vi "hardware_initialize_hardware.vi"(8 "error in (no error)":errorcluster, 11 "tt20 in":refnum<class "tt20.lvclass">) -> (0 "error out":errorcluster, 3 "tt20 out":refnum<class "tt20.lvclass">)   [LabVIEW 2015, in "tt20.lvclass"]
uses:
  tt20.lvclass
  tt20.lvclass/tt20.ctl
  C:/Users/MX-Microscope/Documents/LabVIEW Data/lvoop_campus_2018/Detector_Class/Swabian/time_tagger_vis/TTCSharp32.dll
  time_tagger_vis/TTCSharp32.dll
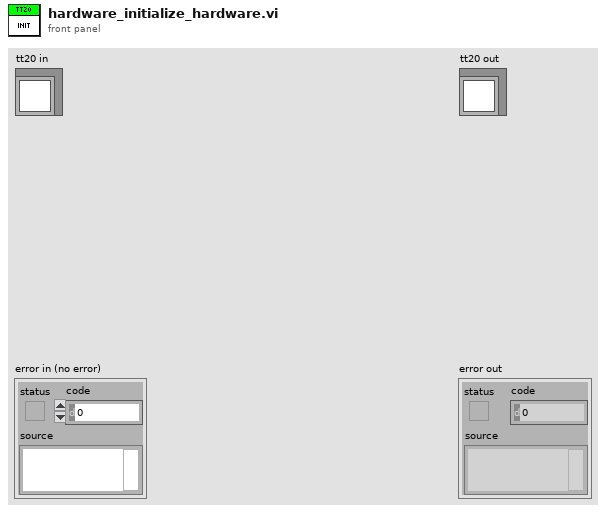
[diagram p1: front panel]
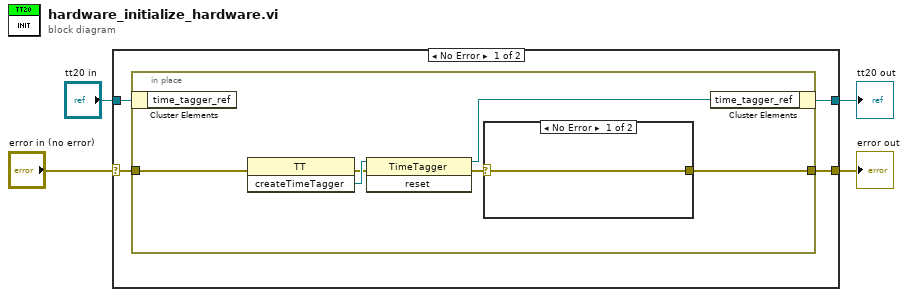
[diagram p0: block diagram]
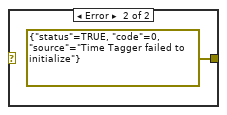
[diagram p2: hidden frame]
diagram:
  n1 = case shown="No Error" "error in (no error)" {
    selector: "error in (no error)" -> [w7 w17]
    tunnel: "tt20 in" -> [w8 w18]
    tunnel: [w6 w17] -> w2
    tunnel: [w5 w18] -> w1
    frame No Error {
      n2 = in-place {
        in-place-border: w7 -> [w14]
        in-place-border: [w11] -> w6
        n3 = in-place-cluster #1(w8) -> ()  [unwired: 1 out]
        n4 = invoke class="TT" method="createTimeTagger"(error in=w14) -> (error out=w12:errorcluster, "createTimeTagger"=w13:refnum<k24>)  [unwired: 2 in, 1 out]
        n5 = invoke class="TimeTagger" method="reset"(reference=w13, error in=w12) -> (reference out=w10:refnum<k24>, error out=w9:errorcluster)  [unwired: 1 in, 1 out]
        n6 = case shown="No Error" w9 {
          selector: w9 -> [w15 _]
          tunnel: [w15 errorcluster {"status"=TRUE, "code"=0, "source"="Time Tagger failed to initialize"} ("error IO")] -> w11
          frame No Error {
          }
          frame Error {
          }
        }
        n7 = in-place-cluster #1("time_tagger_ref"=w10) -> (w5:refnum<class "tt20.lvclass">)
      }
    }
    frame Error {
    }
  }
  "error out" <- w2
  "tt20 out" <- w1
